vi "meters_setup.vi"() -> ()   [LabVIEW 2016]
panel:
  out "Gaussmeter 3 Error":errorcluster
  out "Probe 3 Serial Number":string
  out "Probe 3 Field \nCompensation On":bool
  out "Probe 3\nSensitivity":dbl
  out "Probe 3\nType":u16
  in  "Gaussmeter 3":bool
  in  "VISA Gaussmeter 3":refnum<visa-resource-name>
  out "Gaussmeter 2 Error":errorcluster
  out "Probe 2 Serial Number":string
  out "Probe 2 Field \nCompensation On":bool
  out "Probe 2\nSensitivity":dbl
  out "Probe 2\nType":u16
  in  "Gaussmeter 2":bool
  in  "VISA Gaussmeter 2":refnum<visa-resource-name>
  out "Gaussmeter 1 Error":errorcluster
  out "Probe 1 Serial Number":string
  out "Probe 1 Field \nCompensation On":bool
  out "Probe 1\nSensitivity":dbl
  out "Probe 1\nType":u16
  in  "Gaussmeter 1":bool
  in  "VISA Gaussmeter 1":refnum<visa-resource-name>
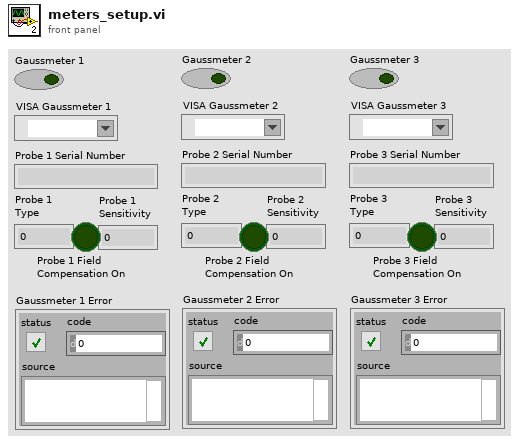
[diagram p1: front panel]
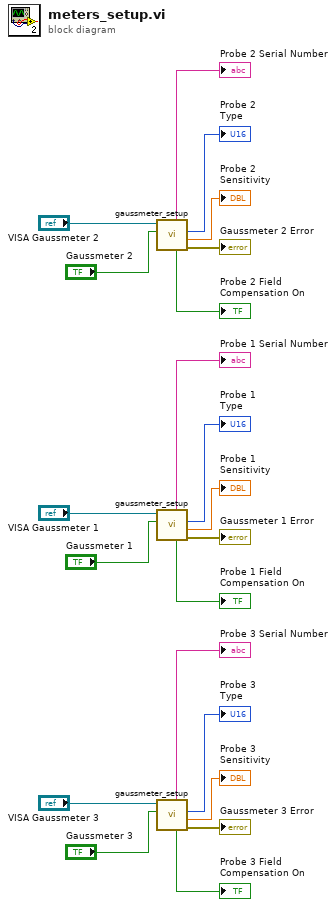
[diagram p0: block diagram]
diagram:
  n1 = call "gaussmeter_setup.vi"("On/Off"="Gaussmeter 2", "VISA Gaussmeter"="VISA Gaussmeter 2") -> ("error out"=→"Gaussmeter 2 Error":errorcluster, "Probe Sensitivity"=→"Probe 2\nSensitivity":dbl, "Probe Type"=→"Probe 2\nType":u16, "Probe Field \nCompensation On"=→"Probe 2 Field \nCompensation On":bool, "Probe Serial Number"=→"Probe 2 Serial Number":string)  [unwired: 4 in, 1 out]
  n2 = call "gaussmeter_setup.vi"("On/Off"="Gaussmeter 1", "VISA Gaussmeter"="VISA Gaussmeter 1") -> ("error out"=→"Gaussmeter 1 Error":errorcluster, "Probe Sensitivity"=→"Probe 1\nSensitivity":dbl, "Probe Type"=→"Probe 1\nType":u16, "Probe Field \nCompensation On"=→"Probe 1 Field \nCompensation On":bool, "Probe Serial Number"=→"Probe 1 Serial Number":string)  [unwired: 4 in, 1 out]
  n3 = call "gaussmeter_setup.vi"("On/Off"="Gaussmeter 3", "VISA Gaussmeter"="VISA Gaussmeter 3") -> ("error out"=→"Gaussmeter 3 Error":errorcluster, "Probe Sensitivity"=→"Probe 3\nSensitivity":dbl, "Probe Type"=→"Probe 3\nType":u16, "Probe Field \nCompensation On"=→"Probe 3 Field \nCompensation On":bool, "Probe Serial Number"=→"Probe 3 Serial Number":string)  [unwired: 4 in, 1 out]
